vi "Trapezoid_Profile_SubVI.vi"(1 "MinFrac_Cruise":dbl=0.3, 2 "Init_Position":dbl, 3 "Vcruise":dbl=200.0, 4 "Deceleration":dbl=100.0, 5 "Acceleration":dbl=100.0, 6 "Final Position":dbl=1000.0) -> (0 "Outputs":T1)   [LabVIEW 2014]
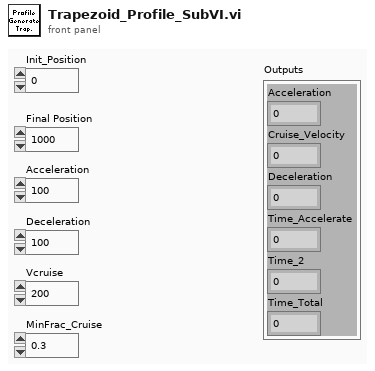
[diagram p1: front panel]
types:
  T1 = cluster{"Acceleration":dbl, "Cruise_Velocity":dbl, "Deceleration":dbl, "Time_Accelerate":dbl, "Time_2":dbl, "Time_Total":dbl}
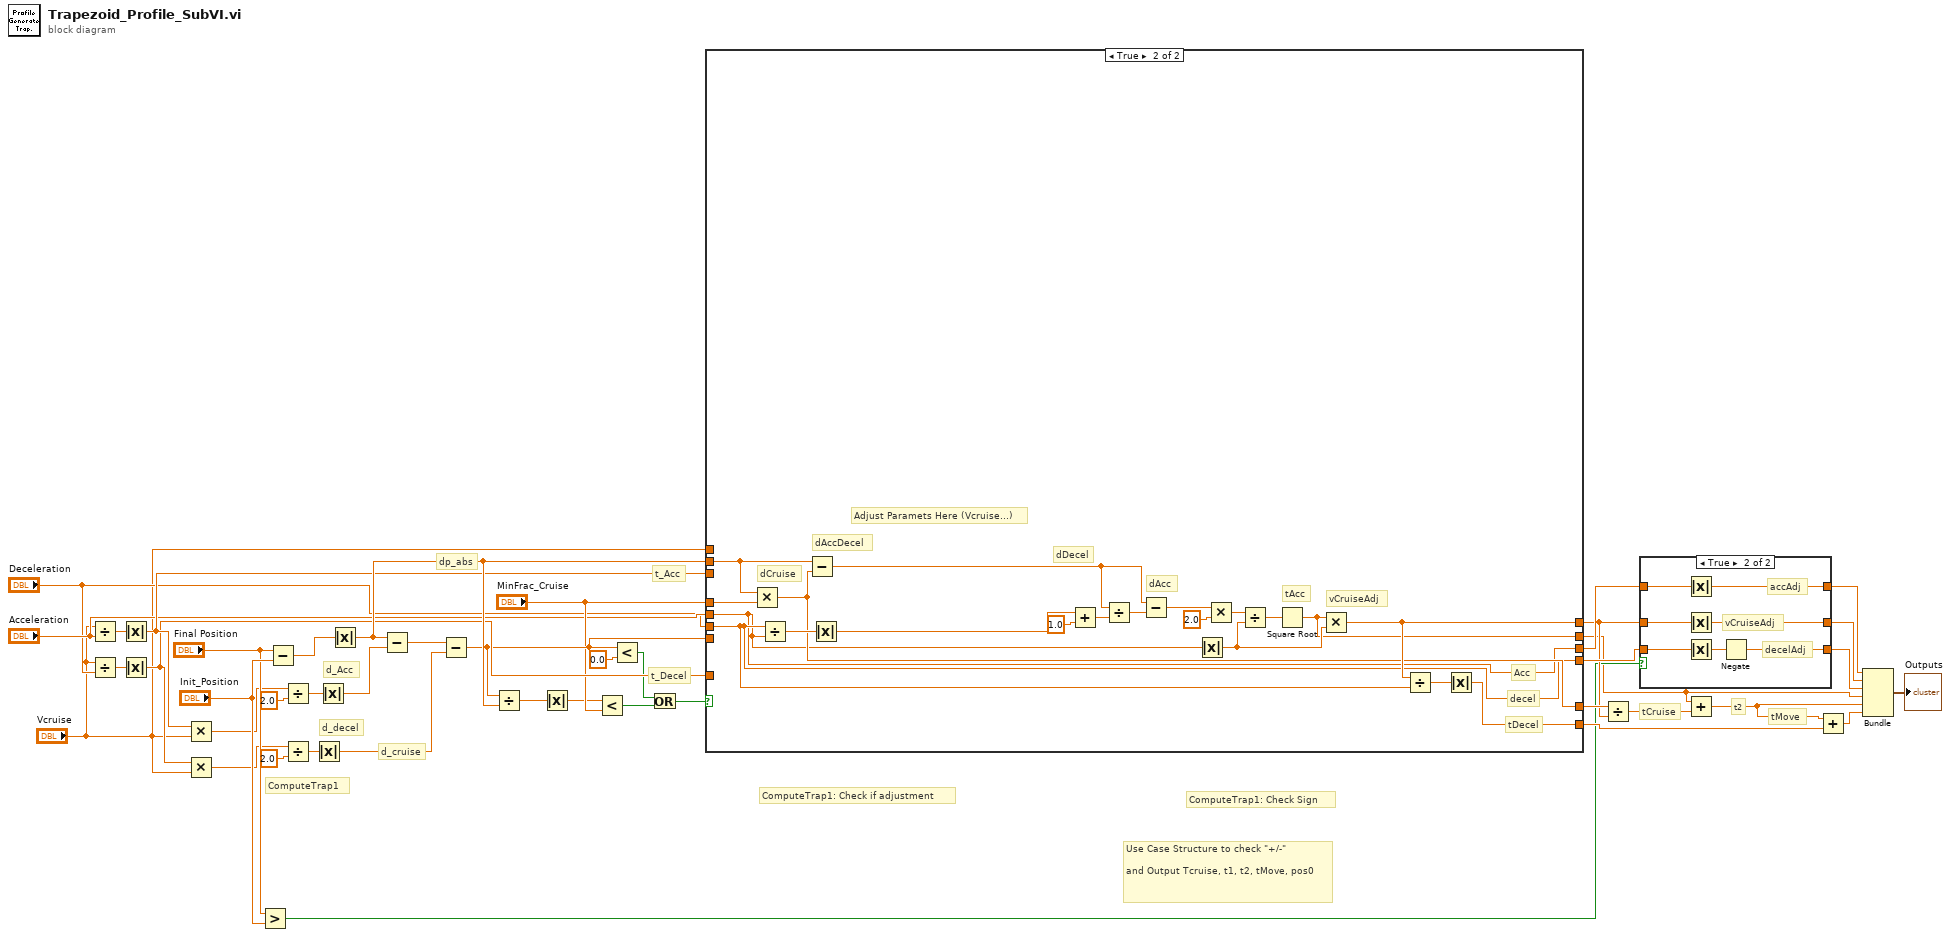
[diagram p0: block diagram]
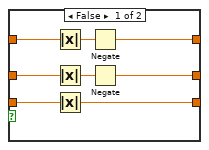
[diagram p2: hidden frame]
diagram:
  # "tMove"
  # "t2"
  # "tCruise"
  # "Use Case Structure to check \"+/-\"\n\nand Output Tcruise, t1, t2, tMove, pos0"
  # "d_cruise"
  # "d_decel"
  # "d_Acc"
  # "t_Decel"
  # "t_Acc"
  # "dp_abs"
  # "ComputeTrap1: Check Sign"
  # "ComputeTrap1: Check if adjustment"
  # "ComputeTrap1"
  n1 = Divide(x="Vcruise", y="Acceleration") -> (x/y=w17:dbl)
  n2 = Divide(x="Vcruise", y="Deceleration") -> (x/y=w18:dbl)
  n3 = Absolute Value(x=w17) -> (abs(x)=w41:dbl)
  n4 = Absolute Value(x=w18) -> (abs(x)=w40:dbl)
  n5 = Multiply(x=w41, y="Vcruise") -> (x*y=w19:dbl)
  n6 = Multiply(x=w40, y="Vcruise") -> (x*y=w24:dbl)
  n7 = Greater?(x="Final Position", y="Init_Position") -> (0:w9:bool)
  n8 = Subtract(x="Final Position", y="Init_Position") -> (x-y=w16:dbl)
  n9 = Divide(x=w19, y=2.0) -> (x/y=w21:dbl)
  n10 = Divide(x=w24, y=2.0) -> (x/y=w22:dbl)
  n11 = Absolute Value(x=w22) -> (abs(x)=w38:dbl)
  n12 = Absolute Value(x=w21) -> (abs(x)=w39:dbl)
  n13 = Absolute Value(x=w16) -> (abs(x)=w42:dbl)
  n14 = Subtract(x=w42, y=w39) -> (x-y=w25:dbl)
  n15 = Subtract(x=w25, y=w38) -> (x-y=w37:dbl)
  n16 = Divide(x=w37, y=w42) -> (x/y=w12:dbl)
  n17 = Absolute Value(x=w12) -> (abs(x)=w11:dbl)
  n18 = Less?(x=w11, y="MinFrac_Cruise") -> (x < y?=w10:bool)
  n19 = Less?(x=w37, y=0.0) -> (x < y?=w13:bool)
  n20 = Or(x=w13, y=w10) -> (x .or. y?=w14:bool)
  n21 = case shown="True" w14 {
    tunnel: "MinFrac_Cruise" -> [_ w68]
    tunnel: w42 -> [_ w67]
    tunnel: "Acceleration" -> [w45 w49]
    tunnel: "Deceleration" -> [w44 w50]
    tunnel: "Vcruise" -> [w48 _]
    tunnel: [w48 w54] -> w29
    tunnel: [w47 w53] -> w3
    tunnel: [w46 w52] -> w30
    tunnel: w41 -> [w47 _]
    tunnel: w37 -> [w46 _]
    tunnel: [w45 w49] -> w32
    tunnel: [w44 w50] -> w31
    tunnel: [w43 w51] -> w26
    tunnel: w40 -> [w43 _]
    frame False {
      # "t_Decel"
      # "Decel"
      # "Acc"
      # "d_Cruise"
      # "t_Acc"
      # "vCruiseAdj"
      # "vCruiseAdj = vCruise"
    }
    frame True {
      # "Acc"
      # "decel"
      # "tDecel"
      # "vCruiseAdj"
      # "tAcc"
      # "dAcc"
      # "dDecel"
      # "dAccDecel"
      # "dCruise"
      # "Adjust Paramets Here (Vcruise...)"
      n22 = Multiply(x=w67, y=w68) -> (x*y=w52:dbl)
      n23 = Divide(x=w50, y=w49) -> (x/y=w66:dbl)
      n24 = Subtract(x=w67, y=w52) -> (x-y=w61:dbl)
      n25 = Absolute Value(x=w66) -> (abs(x)=w65:dbl)
      n26 = Add(x=w65, y=1.0) -> (x+y=w63:dbl)
      n27 = Divide(x=w61, y=w63) -> (x/y=w62:dbl)
      n28 = Subtract(x=w61, y=w62) -> (x-y=w60:dbl)
      n29 = Absolute Value(x=w49) -> (abs(x)=w56:dbl)
      n30 = Multiply(x=w60, y=2.0) -> (x*y=w58:dbl)
      n31 = Divide(x=w58, y=w56) -> (x/y=w57:dbl)
      n32 = Square Root(x=w57) -> (sqrt(x)=w53:dbl)
      n33 = Multiply(x=w53, y=w56) -> (x*y=w54:dbl)
      n34 = Divide(x=w54, y=w50) -> (x/y=w55:dbl)
      n35 = Absolute Value(x=w55) -> (abs(x)=w51:dbl)
    }
  }
  n36 = Divide(x=w30, y=w29) -> (x/y=w8:dbl)
  n37 = case shown="True" w9 {
    tunnel: w32 -> [w76 w83]
    tunnel: w31 -> [w75 w82]
    tunnel: w29 -> [w74 w81]
    tunnel: [w72 w80] -> w6
    tunnel: [w69 w79] -> w5
    tunnel: [w71 w77] -> w4
    frame False {
      n38 = Absolute Value(x=w76) -> (abs(x)=w73:dbl)
      n39 = Absolute Value(x=w74) -> (abs(x)=w70:dbl)
      n40 = Absolute Value(x=w75) -> (abs(x)=w71:dbl)
      n41 = Negate(x=w73) -> (-x=w72:dbl)
      n42 = Negate(x=w70) -> (-x=w69:dbl)
    }
    frame True {
      # "vCruiseAdj"
      # "decelAdj"
      # "accAdj"
      n43 = Absolute Value(x=w83) -> (abs(x)=w80:dbl)
      n44 = Absolute Value(x=w81) -> (abs(x)=w79:dbl)
      n45 = Absolute Value(x=w82) -> (abs(x)=w78:dbl)
      n46 = Negate(x=w78) -> (-x=w77:dbl)
    }
  }
  n47 = Add(x=w3, y=w8) -> (x+y=w2:dbl)
  n48 = Add(x=w2, y=w26) -> (x+y=w1:dbl)
  n49 = Bundle(w6, w5, w4, w3, w2, w1) -> (→"Outputs":cluster{dbl, dbl, dbl, dbl, dbl, dbl})  [unwired: 1 in]
